vi "Prober_ChuckStatusCheck.vi"(8 "error in (no error)":errorcluster, 11 "VeloxTeslaProbestation in":refnum<class "VeloxTeslaProbestation.lvclass">) -> (0 "error out":errorcluster, 2 "Chuck at CONTACT?":bool=TRUE, 3 "VeloxTeslaProbestation out":refnum<class "VeloxTeslaProbestation.lvclass">)   [LabVIEW 2018, in "VeloxTeslaProbestation.lvclass"]
uses:
  VeloxTeslaProbestation.lvclass
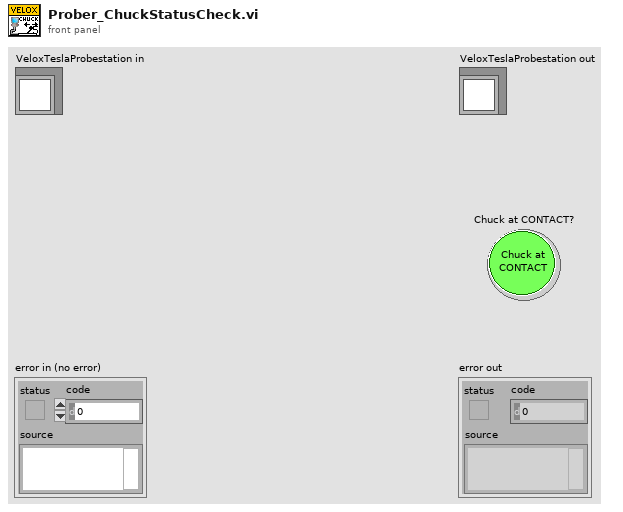
[diagram p1: front panel]
types:
  T1 = cluster{"IsInitialized":cluster{"X axis is initialized":bool, "y axis is initialized":bool, "Z axis is initialized":bool, "Theta axis is initialized":bool}, "Mode":cluster{"Overtravel is enabled":bool, "Auto Z is enabled":bool, "Interlock is enabled":bool, "Auto contact search":bool, "Contact height is set":bool, "Edge sensor interlock":bool, "AutoQuiet is enabled":bool, "Stage lock is enabled":bool}, "OnEndLimit":cluster{"X on positive limit":bool, "X on negative limit":bool, "Y on positive limit":bool, "Y on negative limit":bool, "Z on positive limit":bool, "Z on negative limit":bool, "Theta on positive limit":bool, "Theta on negative limit":bool}, "IsMoving":cluster{"X is moving":bool, "Y is moving":bool, "Z is moving":bool, "Theta is moving":bool}, "Vacuum on?":bool, "Compensation mode":enum8{"None", "Prober", "Offset", "Technology"}, "Z Height":enum8{"Undefined", "Search", "Overtravel", "Alignment", "Separation", "Contact"}, "Load position":cluster{"On load position one":bool, "On load position two":bool}, "lift up?":bool, "Chuck camera":enum8{"Undefined", "On chuck", "At park position"}}
  T2 = enum8{"Undefined", "Search", "Overtravel", "Alignment", "Separation", "Contact"}
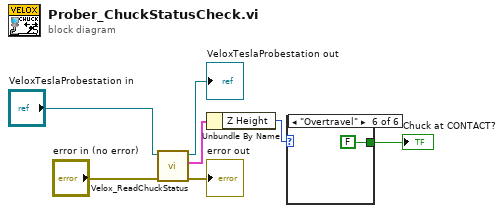
[diagram p0: block diagram]
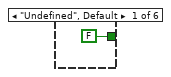
[diagram p2: hidden frame]
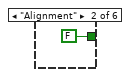
[diagram p3: hidden frame]
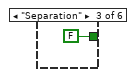
[diagram p4: hidden frame]
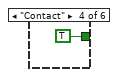
[diagram p5: hidden frame]
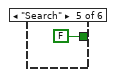
[diagram p6: hidden frame]
diagram:
  n1 = call-dynamic "Velox_ReadChuckStatus.vi"("error in (no error)"="error in (no error)", "VeloxTeslaProbestation in"="VeloxTeslaProbestation in") -> ("error out"=→"error out":errorcluster, "Status"=w5:T1, "VeloxTeslaProbestation out"=→"VeloxTeslaProbestation out":refnum<class "VeloxTeslaProbestation.lvclass">)  [unwired: 7 in]
  n2 = Unbundle By Name(w5) -> ("Z Height"=w4:T2)
  n3 = case shown="\"Overtravel\"" w4 {
    tunnel: [FALSE ("Chuck at CONTACT?") FALSE ("Chuck at CONTACT?") FALSE ("Chuck at CONTACT?") TRUE ("Chuck at CONTACT?") FALSE ("Chuck at CONTACT?") FALSE ("Chuck at CONTACT?")] -> w3
    frame "Undefined", Default {
    }
    frame "Alignment" {
    }
    frame "Separation" {
    }
    frame "Contact" {
    }
    frame "Search" {
    }
    frame "Overtravel" {
    }
  }
  "Chuck at CONTACT?" <- w3
